vi "Forward_t.vi"(8 "error in (no error)":errorcluster, 10 "Time":dbl) -> (0 "error out":errorcluster, 2 "Done":bool)   [LabVIEW 2019]
uses:
  Timer.vi
  Simulated Robot/Simulation SubVIs/Simulation SubVIs.lvlib
panel:
  out "Diff. x Z":dbl
  out "Right":dbl
  out "Left":dbl
  out "Diff.":dbl
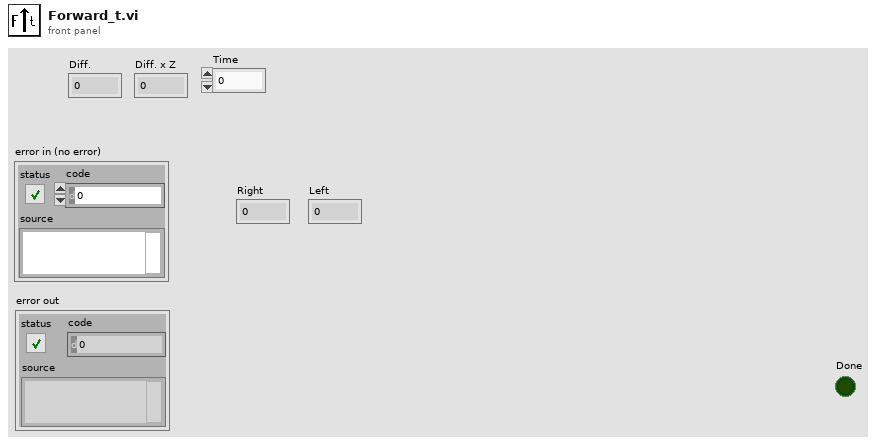
[diagram p1: front panel]
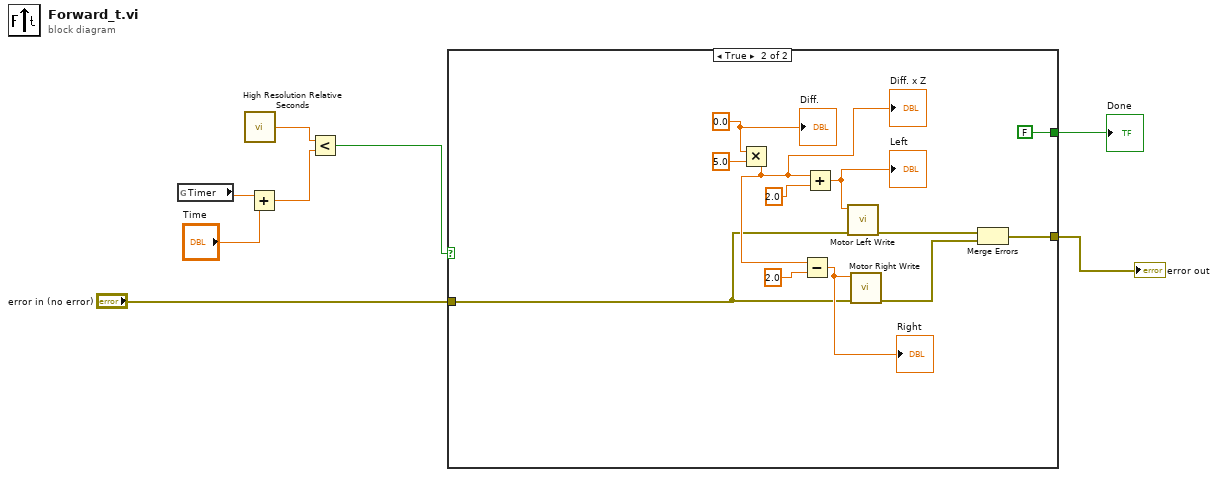
[diagram p0: block diagram]
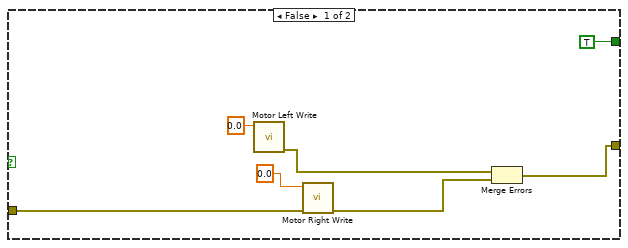
[diagram p2: hidden frame]
diagram:
  n1 = global read "Timer.vi" "Timer"() -> (w5:dbl)
  n2 = call <vilib>:"High Resolution Relative Seconds.vi"() -> ("relative seconds"=w6:dbl)
  n3 = Add(x=w5, y="Time") -> (x+y=w4:dbl)
  n4 = Less?(x=w6, y=w4) -> (x < y?=w1:bool)
  n5 = case shown="True" w1 {
    tunnel: [w11 w18] -> w8
    tunnel: "error in (no error)" -> [w10 w19]
    tunnel: [TRUE ("Done") FALSE ("Done")] -> w7
    frame False {
      n6 = call "Motor Left Write.vi"("left motor ccw velocity (rad/s)"=0.0) -> ("error out"=w15:errorcluster)  [unwired: 10 in]
      n7 = call "Motor Right Write.vi"("error in (no error)"=w10, "right motor ccw velocity (rad/s)"=0.0) -> ("error out"=w14:errorcluster)  [unwired: 9 in]
      n8 = Merge Errors(w15, w14) -> (w11:errorcluster)
    }
    frame True {
      w16 = 0.0 ("x")
      n9 = Multiply(x=w16, y=5.0) -> (x*y=w21:dbl)
      "Diff. x Z" <- w21
      n10 = Subtract(x=w21, y=2.0) -> (x-y=w23:dbl)
      "Right" <- w23
      n11 = Add(x=w21, y=2.0 ("left motor ccw velocity (rad/s)")) -> (x+y=w22:dbl)
      "Left" <- w22
      n12 = call "Motor Left Write.vi"("error in (no error)"=w19, "left motor ccw velocity (rad/s)"=w22) -> ("error out"=w26:errorcluster)  [unwired: 9 in]
      n13 = call "Motor Right Write.vi"("error in (no error)"=w19, "right motor ccw velocity (rad/s)"=w23) -> ("error out"=w27:errorcluster)  [unwired: 9 in]
      n14 = Merge Errors(w26, w27) -> (w18:errorcluster)
      "Diff." <- w16
    }
  }
  "error out" <- w8
  "Done" <- w7
